vi "_PutData_Float.vi"(7 "Index":i32=-1, 8 "Error In":errorcluster, 10 "Data":sgl, 11 "ByteBuffer In":refnum<class "ByteBuffer.lvclass">) -> (0 "Error Out":errorcluster, 3 "ByteBuffer Out":refnum<class "ByteBuffer.lvclass">)   [LabVIEW 2015, in "ByteBuffer.lvclass"]
uses:
  ByteBuffer.lvclass
  ByteBuffer.lvclass/ByteBuffer.ctl
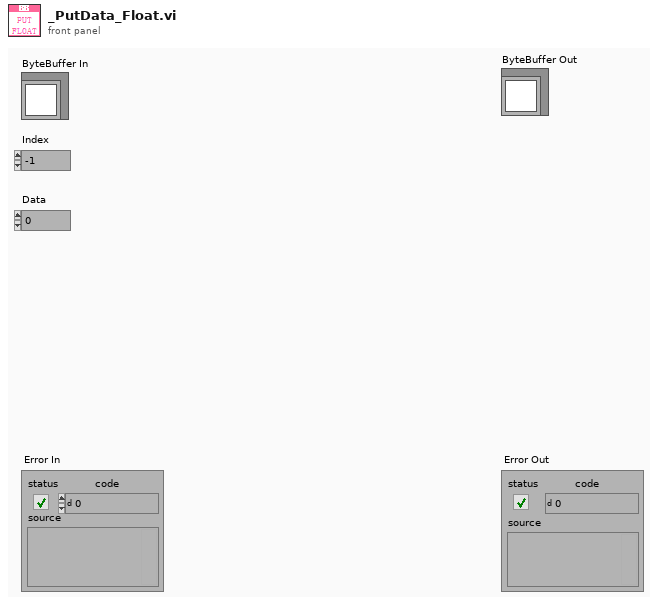
[diagram p1: front panel]
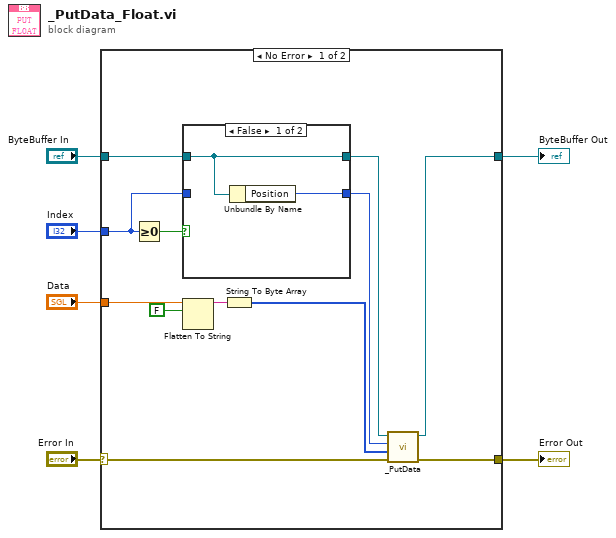
[diagram p0: block diagram]
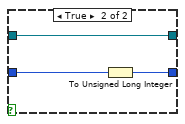
[diagram p2: hidden frame]
diagram:
  n1 = case shown="No Error" "Error In" {
    selector: "Error In" -> [w11 w25]
    tunnel: "ByteBuffer In" -> [w18 w24]
    tunnel: "Index" -> [w16 _]
    tunnel: "Data" -> [w15 _]
    tunnel: [w12 w25] -> w2
    tunnel: [w9 w24] -> w1
    frame No Error {
      n2 = Greater Or Equal To 0?(x=w16) -> (x >= 0?=w17:bool)
      n3 = case shown="False" w17 {
        tunnel: w18 -> [w19 w22]
        tunnel: [w20 w21] -> w8
        tunnel: w16 -> [_ w23]
        tunnel: [w19 w22] -> w10
        frame False {
          n4 = Unbundle By Name(w19) -> ("Position"=w20:u32)
        }
        frame True {
          n5 = To Unsigned Long Integer(number=w23) -> (unsigned 32bit integer=w21:u32)
        }
      }
      n6 = Flatten To String(anything=w15, prepend array or string size? (T)=FALSE) -> (data string=w13:string)  [unwired: 2 in, 2 out]
      n7 = String To Byte Array(string=w13) -> (unsigned byte array=w7:u8[])
      n8 = call "_PutData.vi"("Error In"=w11, "Byte Array"=w7, "Index Or Position"=w8, "ByteBuffer In"=w10) -> ("Error Out"=w12:errorcluster, "ByteBuffer Out"=w9:refnum<class "ByteBuffer.lvclass">)  [unwired: 6 in]
    }
    frame Error {
    }
  }
  "Error Out" <- w2
  "ByteBuffer Out" <- w1
